vi "proccess_annotation_data.vi"(4 "error in":errorcluster, 6 "Annotation Data":string, 7 "Image in":picture) -> (0 "error out":errorcluster, 2 "Annotation data":T1(array[cluster]), 3 "Image out":picture)   [LabVIEW 2019]
doc: "Process the data annotation for camera and draw the bounding box for the objects in the image."
uses:
  controls/annotation.ctl
  <vilib>/regexp/Match Regular Expression.xnode
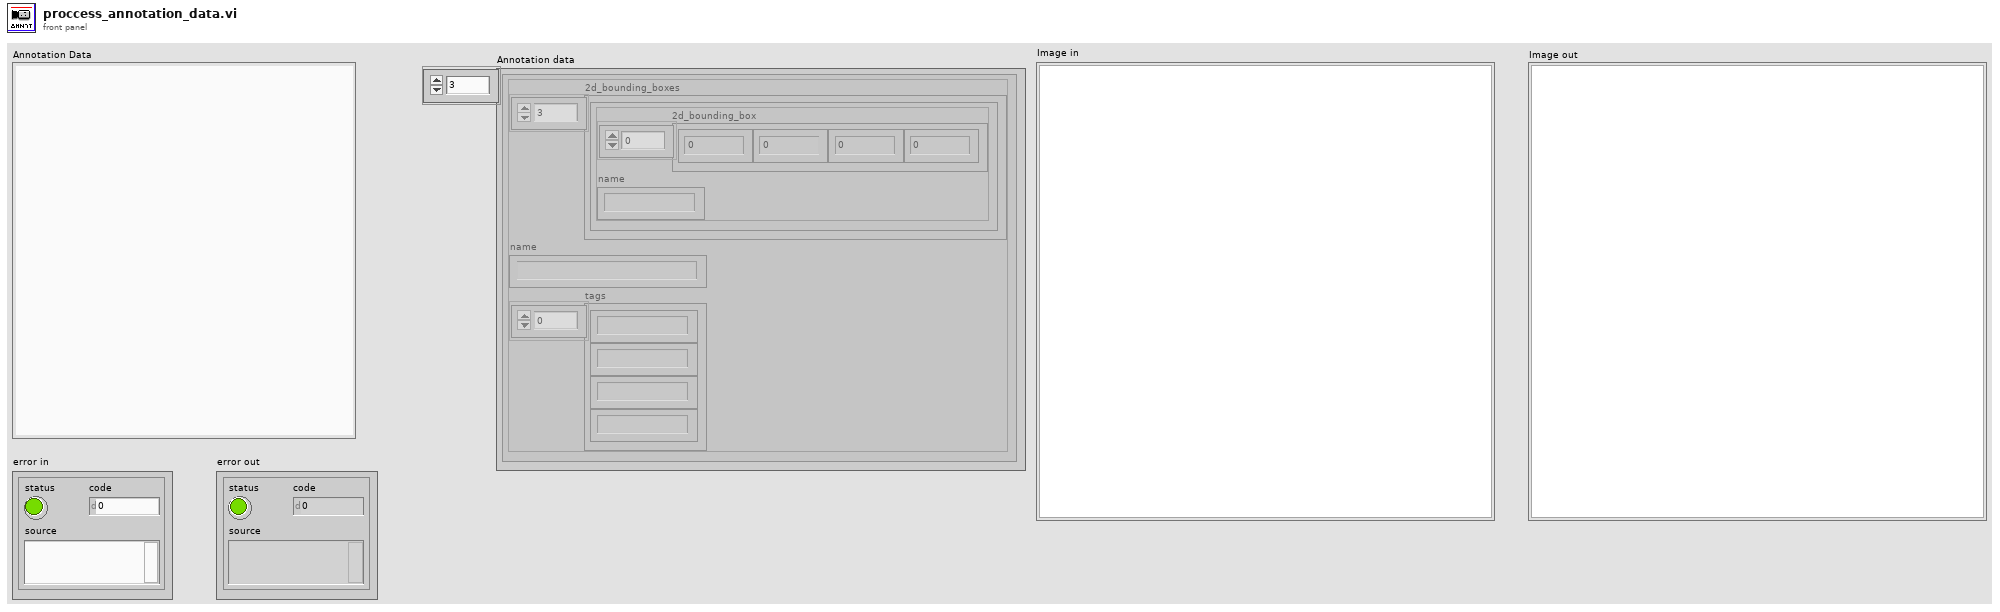
[diagram p1: front panel]
types:
  T1 = cluster{"2d_bounding_boxes":cluster{"2d_bounding_box":dbl[], "name":string}[], "name":string, "tags":string[]}[]
  T2 = typedef "annotation.ctl" = cluster{"actors":cluster{"2d_bounding_boxes":cluster{"2d_bounding_box":dbl[], "name":string}[], "name":string, "tags":string[]}[], "lanes":cluster{"road_id":i64, "lane_id":i64, "s":dbl, "offset":i64, "center":cluster{"x":dbl, "y":dbl}[], "left":cluster{"x":dbl, "y":dbl}[], "right":cluster{"x":dbl, "y":dbl}[]}[]}
  T3 = cluster{"left":i16, "top":i16, "right":i16, "bottom":i16}
  T4 = cluster{"Width":i16, "Style":enum32{"Solid", "Dash", "Dot", "DashDot", "DashDotDot"}}
  T5 = cluster{"2d_bounding_box":dbl[], "name":string}[]
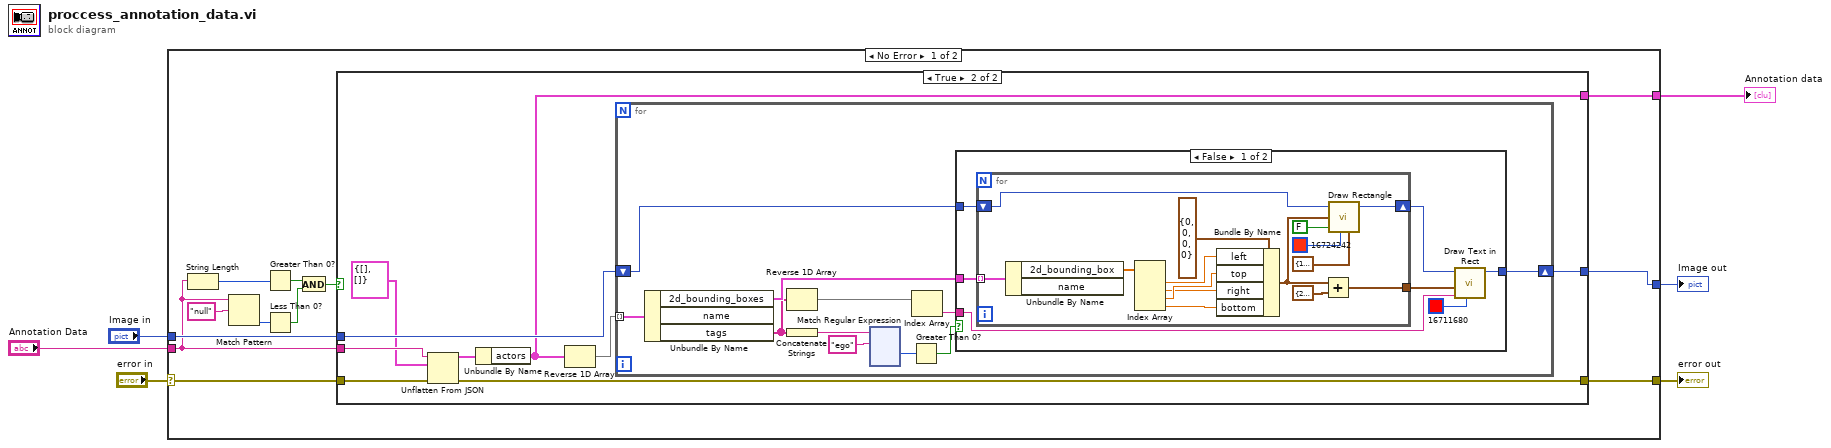
[diagram p0: block diagram]
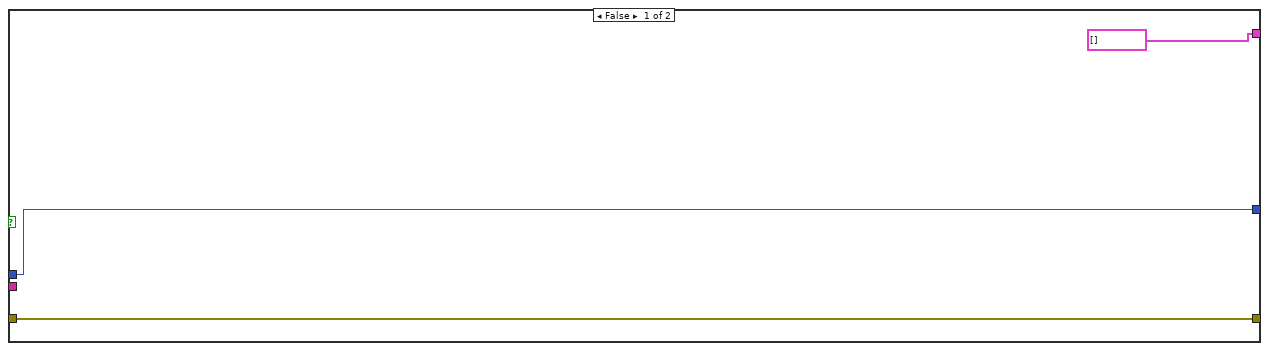
[diagram p2: hidden frame]
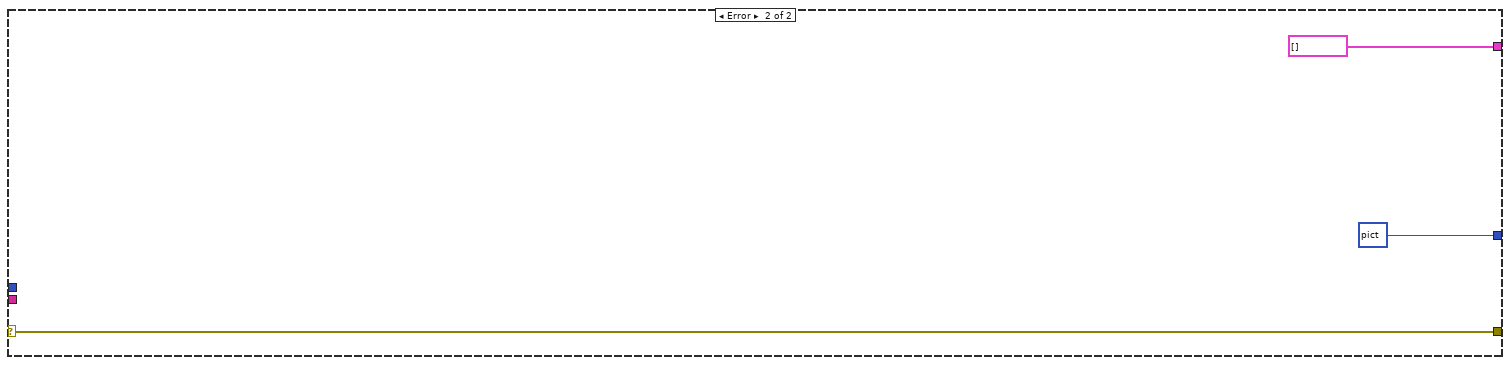
[diagram p4: hidden frame]
diagram:
  n1 = case shown="No Error" "error in" {
    selector: "error in" -> [w18 w181]
    tunnel: [w17 w181] -> w5
    tunnel: [w16 T1 []] -> w4
    tunnel: "Annotation Data" -> [w12 _]
    tunnel: "Image in" -> [w14 _]
    tunnel: [w13 picture data[5B] ("Camera")] -> w1
    frame No Error {
      n2 = String Length(string=w12) -> (length=w15:i32)
      n3 = Match Pattern(string=w12, regular expression="null") -> (offset past match=w8:i32)  [unwired: 1 in, 3 out]
      n4 = Greater Than 0?(x=w15) -> (x > 0?=w9:bool)
      n5 = Less Than 0?(x=w8) -> (x < 0?=w7:bool)
      n6 = And(x=w9, y=w7) -> (x .and. y?=w10:bool)
      n7 = case shown="True" w10 {
        tunnel: w18 -> [w20 w30]
        tunnel: [w20 w28] -> w17
        tunnel: [T1 [] w22] -> w16
        tunnel: w12 -> [_ w29]
        tunnel: w14 -> [w19 w27]
        tunnel: [w19 w26] -> w13
        frame False {
        }
        frame True {
          n8 = Unflatten From JSON(JSON string=w29, type and defaults=T2 {"actors"=[], "lanes"=[]} ("Annotation"), error in (no error)=w30) -> (value=w25:T2, error out=w28:errorcluster)  [unwired: 4 in]
          n9 = Unbundle By Name(w25) -> ("actors"=w22:T1)
          n10 = Reverse 1D Array(array=w22) -> (reversed array=w24:T1)
          n11 = for {
            tunnel: w24 -> [w41] mode=indexing
            shift-right: [w39] -> w26
            shift-left: w27 -> [w36]
            n12 = Unbundle By Name(w41) -> ("2d_bounding_boxes"=w40:T5, "tags"=w32:string[])  [unwired: 1 out]
            n13 = Reverse 1D Array(array=w32) -> (reversed array=w37:string[])
            n14 = Concatenate Strings(w32) -> (w31:string)
            n15 = xnode "Match Regular Expression"("input string"=w31, "regular expression"="ego") -> ("offset past match"=w34:i32)  [unwired: 4 in, 4 out]
            n16 = Greater Than 0?(x=w34) -> (x > 0?=w33:bool)
            n17 = Index Array(array=w37) -> (element=w38:string)  [unwired: 1 in]
            n18 = case shown="False" w33 {
              tunnel: w40 -> [w48 _]
              tunnel: [w45 w64] -> w39
              tunnel: w38 -> [w43 _]
              tunnel: w36 -> [w42 w64]
              frame False {
                n19 = for {
                  tunnel: w48 -> [w63] mode=indexing
                  tunnel: [w51] -> w47
                  shift-right: [w50] -> w46
                  shift-left: w42 -> [w49]
                  n20 = Unbundle By Name(w63) -> ("2d_bounding_box"=w61:dbl[])  [unwired: 1 out]
                  n21 = Index Array(array=w61) -> (element #1=w54:dbl, element #2=w56:dbl, element #3=w57:dbl, element #4=w55:dbl)  [unwired: 4 in]
                  n22 = Bundle By Name(cluster=T3 {"left"=0, "top"=0, "right"=0, "bottom"=0} ("rect"), "left"=w54, "top"=w57, "right"=w56, "bottom"=w55) -> (w53:T3)
                  n23 = Add(x=w53, y=T3 {"left"=25, "top"=-10, "right"=100, "bottom"=10}) -> (x+y=w51:T3)
                  n24 = call <vilib>:"Draw Rectangle.vi"("picture"=w49, "rect"=w53, "fill?(F)"=FALSE, "color(black)"=u32 16724242, "pen"=T4 {"Width"=1, "Style"=enum."DashDotDot"}) -> ("new picture"=w50:picture)  [unwired: 4 in]
                }
                n25 = call <vilib>:"Draw Text in Rect.vi"("text color(black)"=u32 16711680, "text"=w43, "rect"=w47, "picture"=w46) -> ("new picture"=w45:picture)  [unwired: 7 in]
              }
              frame True {
              }
            }
          }
        }
      }
    }
    frame Error {
    }
  }
  "error out" <- w5
  "Annotation data" <- w4
  "Image out" <- w1
